vi "Divider4.vi"() -> (8 "Divider4":refnum<class "Divider4.lvclass">)   [LabVIEW 2017, in "Divider4.lvclass"]
uses:
  Divider4.lvclass
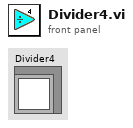
[diagram p1: front panel]
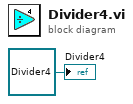
[diagram p0: block diagram]
diagram:
  "Divider4" <- refnum<class "Divider4.lvclass"> refnum ("Divider4.lvclass")
